vi "report.vi"() -> ()   [LabVIEW 2017]
uses:
  <vilib>/addons/database/Connection.llb/DB Tools Open Connec (Path).vi
  <vilib>/Utility/file.llb/Write Delimited Spreadsheet (string).vi
  <vilib>/addons/database/NI_Database_API.lvlib
  Brembo_DOCKING_2017/Source_Code/BREMBO_DOCKING_FOUR/Brembo V3.6_Thrd_m9_v7/GLobal_variable/Login Details.vi
panel:
  in  "delete":bool
  in  "Scan Barcode":bool
  out "error out":errorcluster
  in  "error in (no error)":errorcluster
  in  "FROM":timestamp format="%<%x>T"
  in  "TO":timestamp format="%<%x>T"
  out "table":string[][](table)
  out "Table header":string[](array[string])
  in  "Barcode":string
  in  "Type Wise":enum16{"Barcode Wise", "Datewise"}(ring)=enum."Datewise"
  in  "stop":bool
  in  "Export to Excel":bool
  in  "Get Report":bool
  # "REPORT"
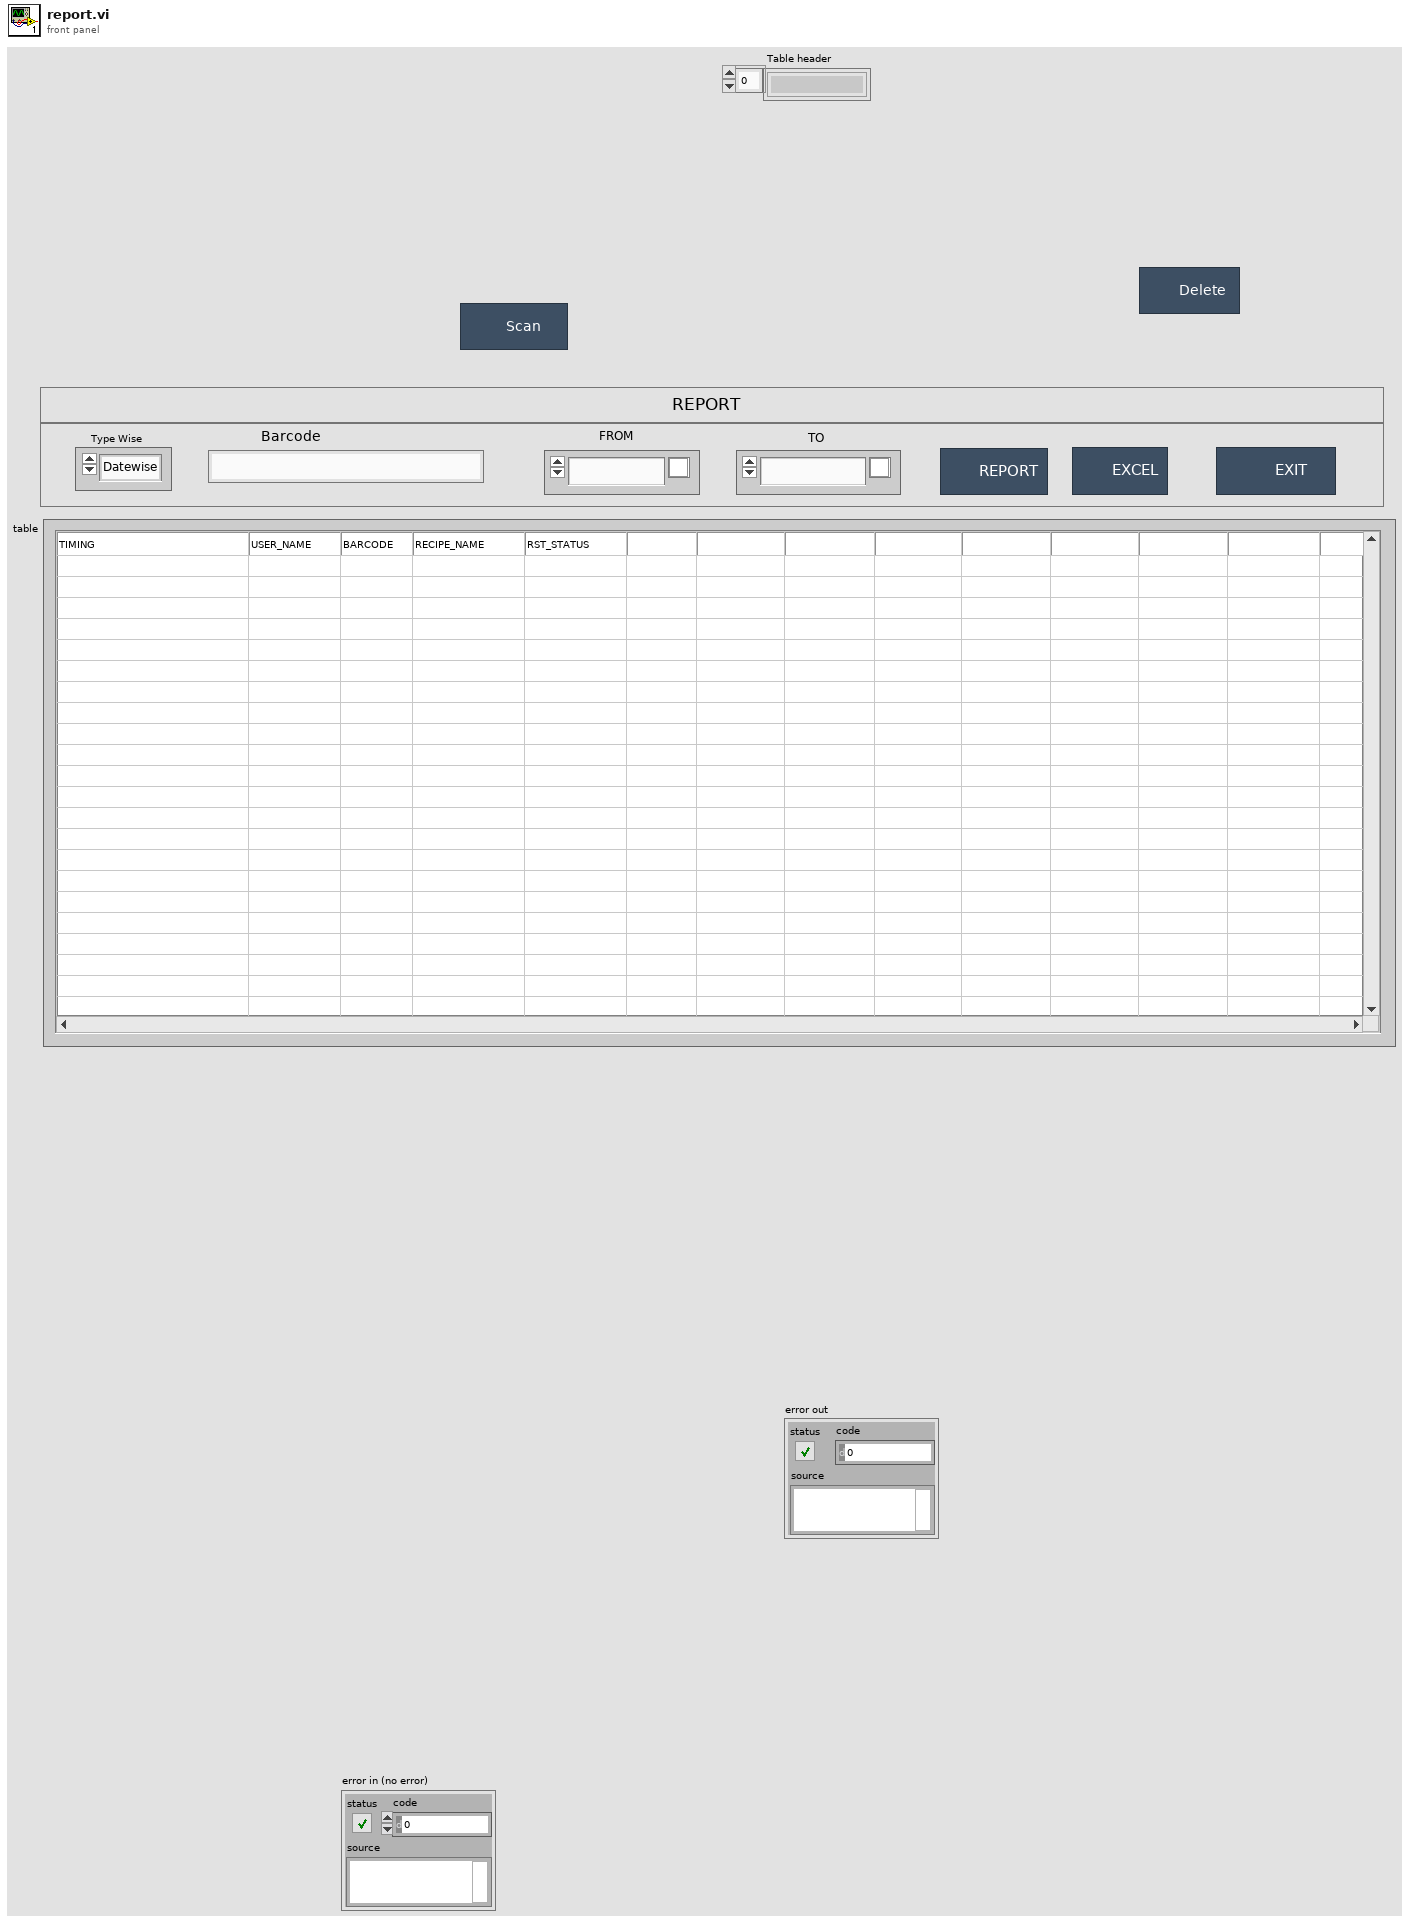
[diagram p1: front panel]
types:
  T1 = typedef "LVDateTimeRec.ctl" = cluster{"fractional second":dbl, "second":i32, "minute":i32, "hour":i32, "day of month":i32, "month":i32, "year":i32, "day of week":i32, "day of year":i32, "DST":i32}
  T2 = typedef "NI_Database_API.lvlib/Conn ObjectReference.ctl" = refnum<k1>
  T3 = enum16{"open", "replace", "create", "open or create", "replace or create", "replace or create with confirmation"}
  T4 = enum32{"invalid app kind", "Development System", "Run Time System", "Student Edition", "Embedded LabVIEW", "Evaluation", "Custom"}
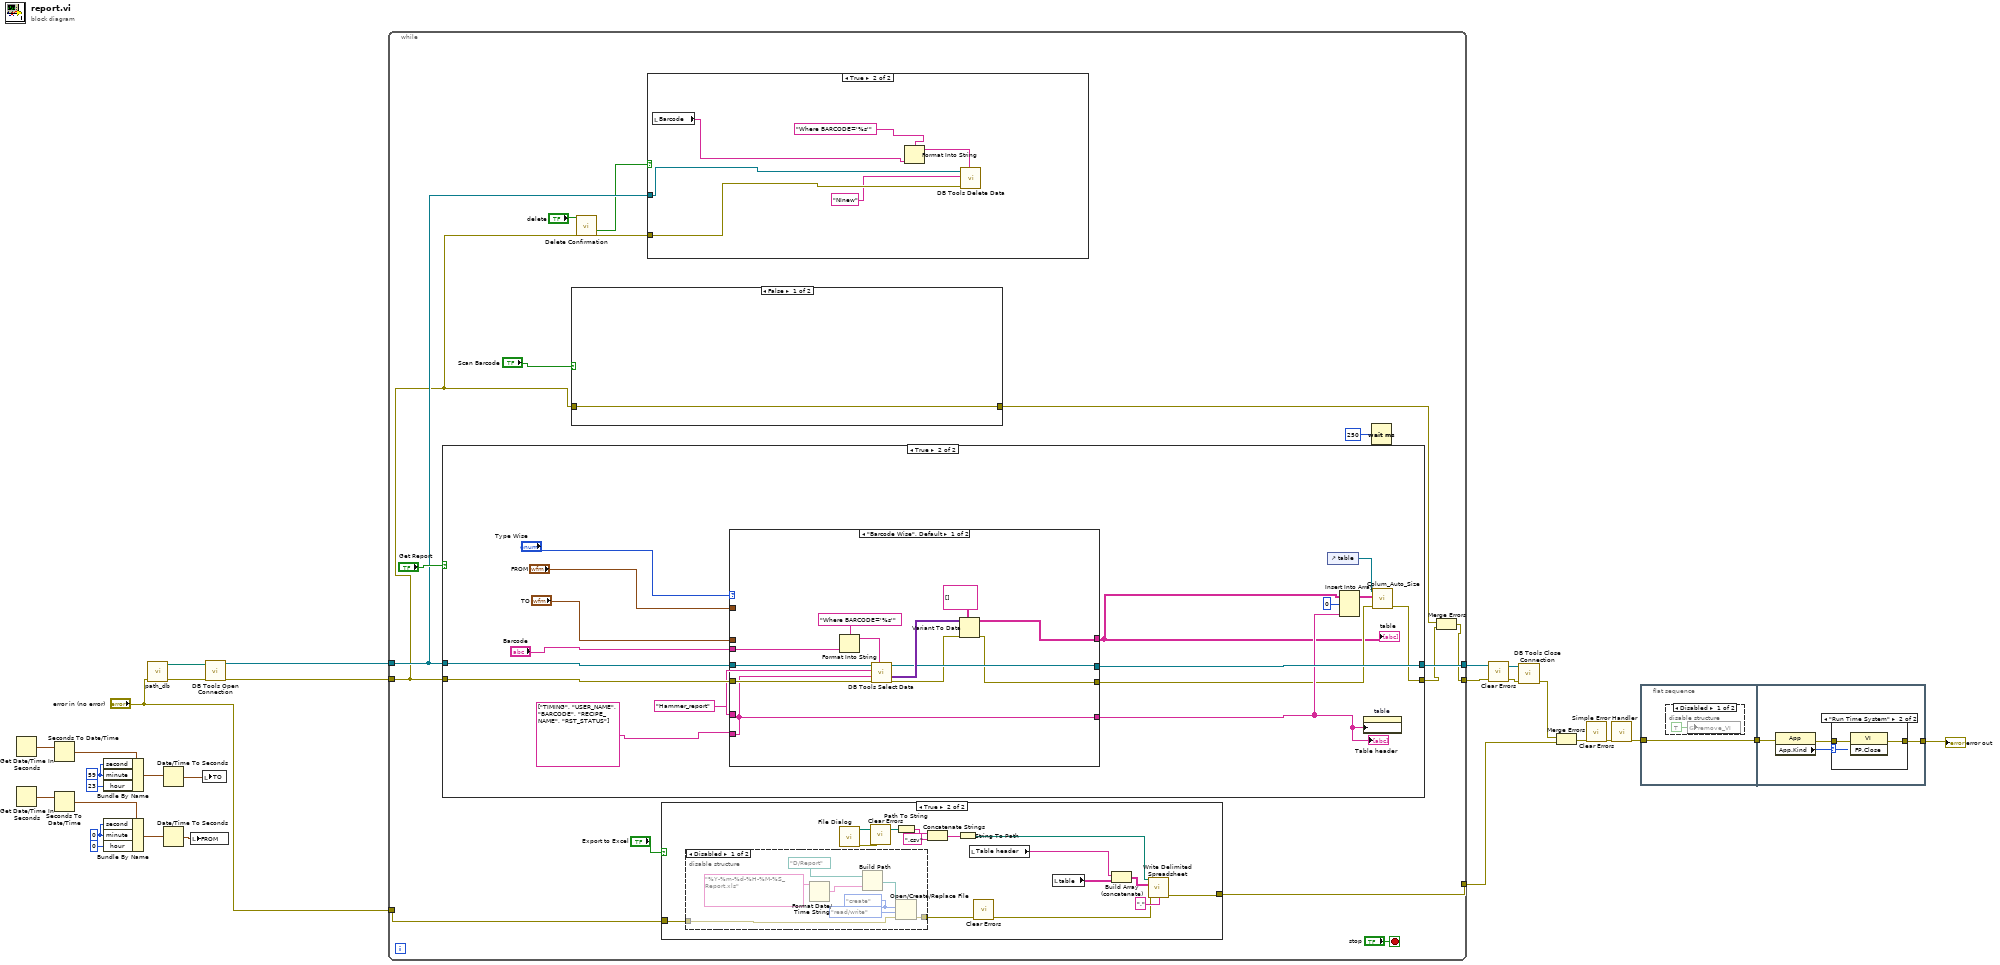
[diagram p0: block diagram]
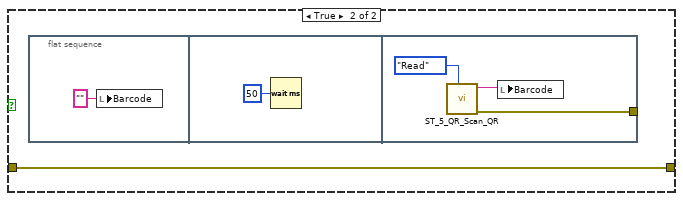
[diagram p5: hidden frame]
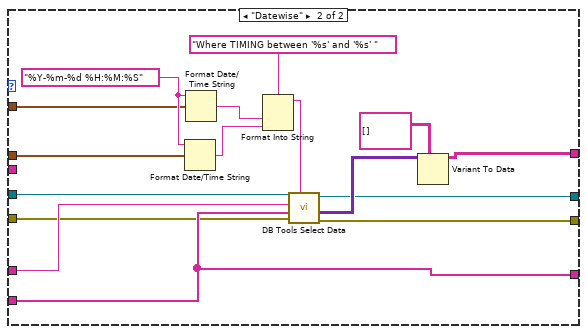
[diagram p9: hidden frame]
diagram:
  w21 = 0 ("minute")
  w22 = 59 ("minute")
  n1 = Get Date/Time In Seconds() -> (seconds since 1Jan1904=w24:timestamp)
  n2 = Get Date/Time In Seconds() -> (seconds since 1Jan1904=w19:timestamp)
  n3 = Seconds To Date/Time(time stamp (now)=w24) -> (date time rec=w25:T1)  [unwired: 1 in]
  n4 = Seconds To Date/Time(time stamp (now)=w19) -> (date time rec=w18:T1)  [unwired: 1 in]
  n5 = Bundle By Name(cluster=w25, "second"=w22, "minute"=w22, "hour"=23) -> (w26:T1)
  n6 = Bundle By Name(cluster=w18, "second"=w21, "minute"=w21, "hour"=0) -> (w17:T1)
  n7 = call "path_db.vi"("error in"="error in (no error)") -> ("error out"=w5:errorcluster, "resulting string"=w6:path)  [unwired: 9 in]
  n8 = Date/Time To Seconds(2:w26) -> (0:w15:timestamp)  [unwired: 1 in]
  n9 = Date/Time To Seconds(2:w17) -> (0:w16:timestamp)  [unwired: 1 in]
  n10 = local write "FROM"(w16) -> ()
  n11 = local write "TO"(w15) -> ()
  n12 = call-poly <vilib>:"DB Tools Open Connection.vi"("error in (no error)"=w5, "connection information"=w6) -> ("error out"=w4:errorcluster, "connection reference"=w8:T2)  [unwired: 6 in]
  n13 = while {
    tunnel: w8 -> [w32]
    tunnel: w4 -> [w31]
    tunnel: [w43] -> w14
    tunnel: [w33] -> w2
    tunnel: "error in (no error)" -> [w41]
    tunnel: [w40] -> w12
    stop <- "stop" stop-if-true
    n14 = case shown="True" "Get Report" {
      tunnel: w32 -> [w81 w96]
      tunnel: w31 -> [w80 w95]
      tunnel: [w81 w94] -> w43
      tunnel: [w80 w88] -> w34
      frame False {
      }
      frame True {
        n15 = case shown="\"Barcode Wise\", Default" "Type Wise" {
          tunnel: w96 -> [w110 w126]
          tunnel: w95 -> [w109 w111]
          tunnel: string[] ["TIMING", "USER_NAME", "BARCODE", "RECIPE_NAME", "RST_STATUS"] -> [w98 w114]
          tunnel: "Hammer_report" ("table") -> [w104 w123]
          tunnel: [w103 w122] -> w94
          tunnel: [w101 w121] -> w84
          tunnel: [w100 w115] -> w82
          tunnel: [w98 w114] -> w90
          tunnel: "Barcode" -> [w99 _]
          tunnel: "FROM" -> [_ w113]
          tunnel: "TO" -> [_ w112]
          frame "Barcode Wise", Default {
            n16 = Format Into String(format string="Where BARCODE='%s'", w99) -> (resulting string=w107:string)  [unwired: 2 in, 1 out]
            n17 = call <vilib>:"DB Tools Select Data.vi"("condition"=w107, "error in (no error)"=w109, "columns"=w98, "table"=w104, "connection reference"=w110) -> ("error out"=w102:errorcluster, "data"=w106:variant[][], "connection reference out"=w103:T2)  [unwired: 1 in]
            n18 = Variant To Data(error in=w102, type=string[][] [], Variant=w106) -> (data=w100:string[][], error out=w101:errorcluster)
          }
          frame "Datewise" {
            w117 = "%Y-%m-%d %H:%M:%S" ("time format string (%c)")
            n19 = Format Date/Time String(time format string (%c)=w117, seconds (now)=w112) -> (date/time string=w118:string)  [unwired: 1 in]
            n20 = Format Date/Time String(time format string (%c)=w117, seconds (now)=w113) -> (date/time string=w119:string)  [unwired: 1 in]
            n21 = Format Into String(format string="Where TIMING between '%s' and '%s' ", w119, w118) -> (resulting string=w120:string)  [unwired: 2 in, 1 out]
            n22 = call <vilib>:"DB Tools Select Data.vi"("condition"=w120, "error in (no error)"=w111, "columns"=w114, "table"=w123, "connection reference"=w126) -> ("error out"=w121:errorcluster, "data"=w125:variant[][], "connection reference out"=w122:T2)  [unwired: 1 in]
            n23 = Variant To Data(type=string[][] [], Variant=w125) -> (data=w115:string[][])  [unwired: 1 in, 1 out]
          }
        }
        "table" <- w82
        "Table header" <- w90
        n24 = control-ref of="table"() -> (w87:refnum<vi>)
        n25 = Insert Into Array(array=w82, index (row)=0, new element=w90) -> (w86:string[][])  [unwired: 1 in]
        n26 = property on="table" class="Tbl (strict)"("Column Headers[]"=w90) -> ()  [unwired: 2 in, 2 out]
        n27 = call "Colum_Auto_Size.vi"("error in (no error)"=w84, "Table With header"=w86, "Table reference"=w87) -> ("error out"=w88:errorcluster)  [unwired: 8 in]
      }
    }
    n28 = case shown="False" "Scan Barcode" {
      tunnel: w31 -> [w50 w51]
      tunnel: [w50 w51] -> w35
      frame False {
      }
      frame True {
        n29 = flat-sequence {
          tunnel: [w54] -> _
          frame #0 {
            n30 = local write "Barcode"("" ("Barcode")) -> ()
          }
          frame #1 {
            n31 = Wait (ms)(milliseconds to wait=u32 50) -> ()  [unwired: 1 out]
          }
          frame #2 {
            n32 = call "ST_5_QR_Scan_QR.vi"("Enum"=enum16{"Read", "Write"}."Read") -> ("error out"=w54:errorcluster, "LB QR ST 5"=w56:string)  [unwired: 9 in]
            n33 = local write "Barcode"(w56) -> ()
          }
        }
      }
    }
    n34 = call "Delete Confirmation"("Enable"="delete", "error in (no error)"=w31) -> ("OK"=w28:bool, "error out"=w30:errorcluster)  [unwired: 16 in]
    n35 = case shown="True" w28 {
      tunnel: w32 -> [_ w49]
      tunnel: w30 -> [_ w48]
      frame False {
      }
      frame True {
        n36 = local read "Barcode"() -> (w47:string)
        n37 = Format Into String(format string="Where BARCODE='%s'", w47) -> (resulting string=w46:string)  [unwired: 2 in, 1 out]
        n38 = call <vilib>:"DB Tools Delete Data.vi"("condition"=w46, "error in (no error)"=w48, "table"="NInew", "connection reference"=w49) -> ()  [unwired: 6 in, 2 out]
      }
    }
    n39 = case shown="True" "Export to Excel" {
      tunnel: w41 -> [w57 w71]
      tunnel: [w57 w70] -> w40
      frame False {
      }
      frame True {
        n40 = disable-structure shown="Disabled" {
          disable-tunnel: w71 -> [w75 w79]
          disable-tunnel: [w74 w79] -> w59
          frame Disabled {
            w72 = enum16{"read/write", "read-only", "write-only"}."read/write" ("access (0:read/write)")
            w72 = T3."create" ("operation (0:open)")
            n41 = Format Date/Time String(time format string (%c)="%Y-%m-%d-%H-%M-%S_Report.xls") -> (date/time string=w78:string)  [unwired: 2 in]
            n42 = Build Path(base path=path "D:/Report", name or relative path=w78) -> (appended path=w76:path)
            n43 = Open/Create/Replace File(file path (use dialog)=w76, error in=w75, operation (0:open)=w72, access (0:read/write)=w72) -> (error out=w74:errorcluster)  [unwired: 2 in, 2 out]
          }
          frame Enabled {
          }
        }
        n44 = call "File Dialog"() -> ("selected path"=w64:path, "error out"=w65:errorcluster)  [unwired: 12 in, 2 out]
        n45 = call <vilib>:"Clear Errors.vi"("error in (no error)"=w65) -> ()  [unwired: 5 in, 2 out]
        n46 = Path To String(path=w64) -> (string=w63:string)
        n47 = Concatenate Strings(w63, ".csv" ("string")) -> (w61:string)
        n48 = String To Path(string=w61) -> (path=w60:path)
        n49 = local read "Table header"() -> (w67:string[])
        n50 = call <vilib>:"Clear Errors.vi"("error in (no error)"=w59) -> ("error out"=w58:errorcluster)  [unwired: 5 in, 1 out]
        n51 = local read "table"() -> (w68:string[][])
        n52 = Build Array (concatenate)(w67, w68) -> (w69:string[][])
        n53 = call-poly <vilib>:"Write Delimited Spreadsheet.vi"("file path (dialog if empty)"=w60, "2D data"=w69, "error in (no error)"=w58, "delimiter (\\t)"="," ("delimiter (\\t)")) -> ("error out"=w70:errorcluster)  [unwired: 10 in, 1 out]
      }
    }
    n54 = Wait (ms)(milliseconds to wait=u32 250) -> ()  [unwired: 1 out]
    n55 = Merge Errors(w35, w34) -> (w33:errorcluster)
  }
  n56 = call <vilib>:"Clear Errors.vi"("error in (no error)"=w2) -> ("error out"=w1:errorcluster)  [unwired: 5 in, 1 out]
  n57 = call <vilib>:"DB Tools Close Connection.vi"("error in (no error)"=w1, "connection reference"=w14) -> ("error out"=w13:errorcluster)  [unwired: 5 in]
  n58 = Merge Errors(w13, w12) -> (w11:errorcluster)
  n59 = call <vilib>:"Clear Errors.vi"("error in (no error)"=w11) -> ("error out"=w10:errorcluster)  [unwired: 5 in, 1 out]
  n60 = call <vilib>:"Simple Error Handler.vi"("error in (no error)"=w10) -> ("error out"=w9:errorcluster)  [unwired: 4 in, 4 out]
  n61 = flat-sequence {
    tunnel: w9 -> [w127]
    tunnel: [w127] -> w27
    tunnel: w27 -> [w130]
    tunnel: [w129] -> w7
    frame #0 {
      n62 = disable-structure shown="Disabled" {
        frame Disabled {
          n63 = global write "Login Details.vi" "remove_VI"(TRUE ("remove_VI")) -> ()
        }
        frame Enabled {
        }
      }
    }
    frame #1 {
      n64 = property class="App"(error in=w130) -> (error out=w131:errorcluster, "App.Kind"=w132:T4)  [unwired: 1 in, 1 out]
      n65 = case shown="\"Run Time System\"" w132 {
        tunnel: w131 -> [w133 w135]
        tunnel: [w133 w134] -> w129
        frame Default {
        }
        frame "Run Time System" {
          n66 = invoke class="VI" method="FP.Close"(error in=w135) -> (error out=w134:errorcluster)  [unwired: 2 in, 2 out]
        }
      }
    }
  }
  "error out" <- w7
